vi "fgv_simple-counter.vi"(7 "cmd":T1, 8 "error in":errorcluster, 11 "position":i32) -> (0 "error out":errorcluster, 3 "count n":i32)   [LabVIEW 2018]
uses:
  Ctrl/simple counter.ctl
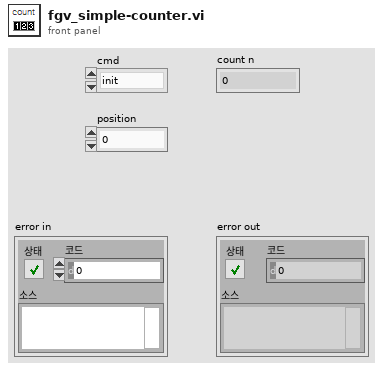
[diagram p1: front panel]
types:
  T1 = typedef "simple counter.ctl" = enum16{"init", "pause", "plus 1", "set", "check"}
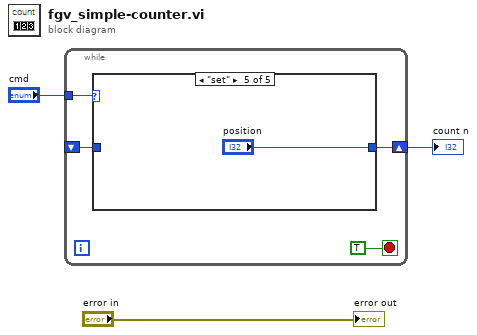
[diagram p0: block diagram]
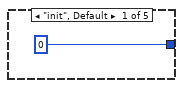
[diagram p2: hidden frame]
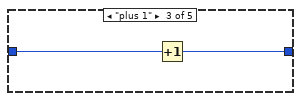
[diagram p4: hidden frame]
diagram:
  n1 = while {
    tunnel: "cmd" -> [w6]
    shift-right: [w5] -> w2
    shift-left: _ -> [w4]
    stop <- TRUE stop-if-true
    n2 = case shown="\"set\"" w6 {
      tunnel: [0 w9 w10 w12 "position"] -> w5
      tunnel: w4 -> [_ w9 w11 w12 _]
      frame "init", Default {
      }
      frame "pause" {
      }
      frame "plus 1" {
        n3 = Increment(x=w11) -> (x+1=w10:i32)
      }
      frame "check" {
      }
      frame "set" {
      }
    }
  }
  "count n" <- w2
  "error out" <- "error in"
